vi "Configure Glitch Trigger Source [GT] Core.vi"(0 "IVI_Scope in":refnum<class "IVI_Scope.lvclass">, 1 "trigger source (\"CHANNEL1\")":string(combo)="CHANNEL1", 2 "trigger level (0.0 V)":dbl[unit] format="%.3f", 3 "glitch width (10 ms)":dbl[unit]=1e-05 format="%^.2e", 4 "glitch polarity (Positive)":i32(ring)=1 items=["Positive"=1, "Negative"=2, "Either"=3], 5 "error in (no error)":errorcluster, 6 "glitch condition (Less Than)":i32(ring)=1 items=["Less Than"=1, "Greater Than"=2]) -> (14 "IVI_Scope out":refnum<class "IVI_Scope.lvclass">, 19 "error out":errorcluster)   [LabVIEW 2015, in "IVI_Scope.lvlib" / "IVI_Scope.lvclass"]
doc: "This VI configures the glitch trigger. A glitch trigger occurs when the trigger signal has a pulse with a width that is less than or greater than the glitch width. You specifiy which comparison criterion to use with the glitchCondition parameter. You specifiy the glitch width in the glitchWidth parameter. You specifiy the polarity of the pulse with the glitchPolarity parameter. The trigger does not actually occur until the edge of a pulse that corresponds to the glitchWidth and glitchPolarity crosses the threshold the end-user specifies in the triggerLevel parameter.\n\nNote:\nThis VI affects instrument behavior only if the trigger type is IVISCOPE_VAL_GLITCH_TRIGGER. Call the IviScope Configure Trigger and IviScope Configure Trigger Coupling VIs to set the trigger type and trigger coupling before calling this VI."
uses:
  IVI_Scope.lvclass
  IVI_Scope.lvclass/IVI_Scope.ctl
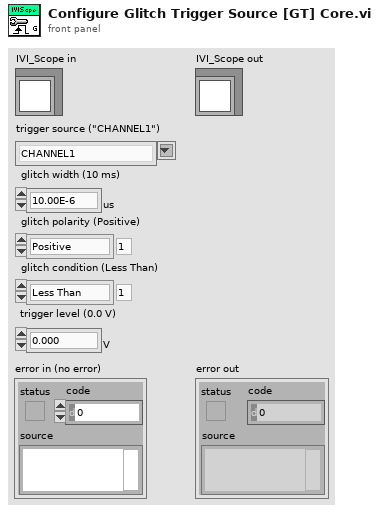
[diagram p1: front panel]
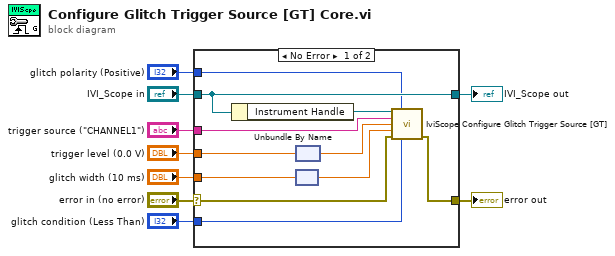
[diagram p0: block diagram]
diagram:
  n1 = case shown="No Error" "error in (no error)" {
    selector: "error in (no error)" -> [w18 w22]
    tunnel: [w17 w22] -> w8
    tunnel: [w20 w21] -> w6
    tunnel: "IVI_Scope in" -> [w20 w21]
    tunnel: "trigger source (\"CHANNEL1\")" -> [w16 _]
    tunnel: "trigger level (0.0 V)" -> [w15 _]
    tunnel: "glitch width (10 ms)" -> [w14 _]
    tunnel: "glitch polarity (Positive)" -> [w13 _]
    tunnel: "glitch condition (Less Than)" -> [w12 _]
    frame No Error {
      n2 = Unbundle By Name(w20) -> ("Instrument Handle"=w19:refnum<k15>)
      n3 = node(w15) -> (w11:dbl)
      n4 = node(w14) -> (w10:dbl)
      n5 = call <vilib>:"IviScope Configure Glitch Trigger Source [GT].vi"("instrument handle"=w19, "glitch polarity (Positive)"=w13, "trigger source (\"CHANNEL1\")"=w16, "trigger level (0.0 V)"=w11, "glitch width (10 ms)"=w10, "error in (no error)"=w18, "glitch condition (Less Than)"=w12) -> ("error out"=w17:errorcluster)  [unwired: 7 in, 1 out]
    }
    frame Error {
    }
  }
  "error out" <- w8
  "IVI_Scope out" <- w6
